vi "Cowl_Execute.vi"() -> ()   [LabVIEW 2019]
uses:
  Cowl_Globals.vi
  Utility_VIs/Basic_Motor_Modes.ctl
  Cowl_States.ctl
  Cowl_Cluster.ctl
panel:
  out "Cowl_Output":dbl
  in  "Kp":dbl
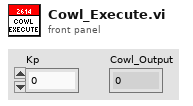
[diagram p1: front panel]
types:
  T1 = typedef "Cowl_Cluster.ctl" = cluster{"Control_State\n":T2, "Manual_Cowl_%Power":dbl}
  T2 = typedef "Cowl_States.ctl" = enum16{"Manual_%VBus", "GoToAngle"}
  T3 = typedef "Basic_Motor_Modes.ctl" = enum16{"Percent_Voltage", "Speed_Control", "Position_Control", "Current"}
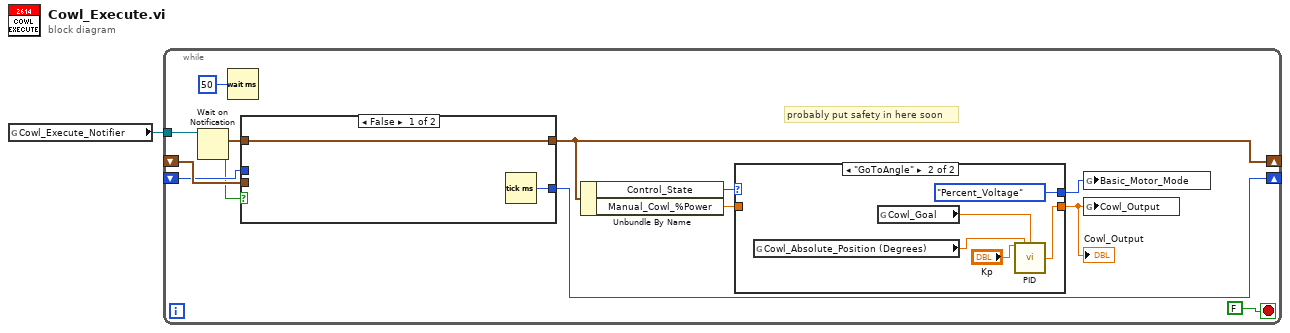
[diagram p0: block diagram]
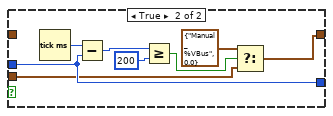
[diagram p2: hidden frame]
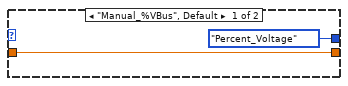
[diagram p3: hidden frame]
diagram:
  n1 = global read "Cowl_Globals.vi" "Cowl_Execute_Notifier"() -> (w1:refnum<notifier>)
  n2 = while {
    tunnel: w1 -> [w12]
    shift-right: [w4] -> _
    shift-left: _ -> [w5]
    shift-right: [w7] -> _
    shift-left: _ -> [w3]
    stop <- FALSE stop-if-true
    # "probably put safety in here soon"
    n3 = Wait on Notification(notifier=w12) -> (notification=w6:T1, timed out?=w2:bool)  [unwired: 3 in, 2 out]
    n4 = Wait (ms)(milliseconds to wait=u32 50) -> ()  [unwired: 1 out]
    n5 = case shown="False" w2 {
      tunnel: w6 -> [w16 _]
      tunnel: [w16 w19] -> w4
      tunnel: [w15 w23] -> w7
      tunnel: w3 -> [_ w23]
      tunnel: w5 -> [_ w18]
      frame False {
        n6 = Tick Count (ms)() -> (millisecond timer value=w15:u32)
      }
      frame True {
        n7 = Tick Count (ms)() -> (millisecond timer value=w24:u32)
        n8 = Subtract(x=w24, y=w23) -> (x-y=w22:u32)
        n9 = Greater Or Equal?(x=w22, y=u32 200) -> (x >= y?=w20:bool)
        n10 = Select(t=T1 {"Control_State\n"=enum."Manual_%VBus", "Manual_Cowl_%Power"=0.0} ("notification"), s=w20, f=w18) -> (s? t:f=w19:T1)
      }
    }
    n11 = Unbundle By Name(w4) -> ("Control_State"=w11:T2, "Manual_Cowl_%Power"=w10:dbl)
    n12 = case shown="\"GoToAngle\"" w11 {
      tunnel: w10 -> [w26 _]
      tunnel: [w26 w31] -> w9
      tunnel: [Basic_Motor_Modes."Percent_Voltage" ("Basic_Motor_Mode") Basic_Motor_Modes."Percent_Voltage" ("Basic_Motor_Mode")] -> w8
      frame "Manual_%VBus", Default {
      }
      frame "GoToAngle" {
        n13 = global read "Cowl_Globals.vi" "Cowl_Absolute_Position (Degrees)"() -> (w28:dbl)
        n14 = global read "Cowl_Globals.vi" "Cowl_Goal"() -> (w29:dbl)
        n15 = call "PID.vi"("Kp"="Kp", "Process Variable"=w28, "Goal"=w29) -> ("Command"=w31:dbl)  [unwired: 10 in, 2 out]
      }
    }
    "Cowl_Output" <- w9
    n16 = global write "Cowl_Globals.vi" "Basic_Motor_Mode"(w8) -> ()
    n17 = global write "Cowl_Globals.vi" "Cowl_Output"(w9) -> ()
  }
